vi "RSNRPZ Configure Statistics Scale.vi"(6 "Range (50.0)":dbl=50.0 format="%^.3e", 7 "Points (200)":i32=200, 8 "error in (no error)":errorcluster, 9 "Reference Level (-30.0 dB)":dbl=-30.0 format="%^.3e", 10 "Channel (1)":i32=1, 11 "VISA session":refnum<visa-resource-name> caption="VISA resource name") -> (0 "error out":errorcluster, 3 "dup VISA session":refnum<visa-resource-name> caption="VISA resource name")   [LabVIEW 2010]
doc: "This VI sets the X-Axis of statistical measurement.\n\nRemote-control command(s):\nSENSe:STATistics:SCALE:X:RLEVel\nSENSe:STATistics:SCALE:X:RANGe\nSENSe:STATistics:SCALE:X:POINts"
uses:
  rsnrpz_32.dll
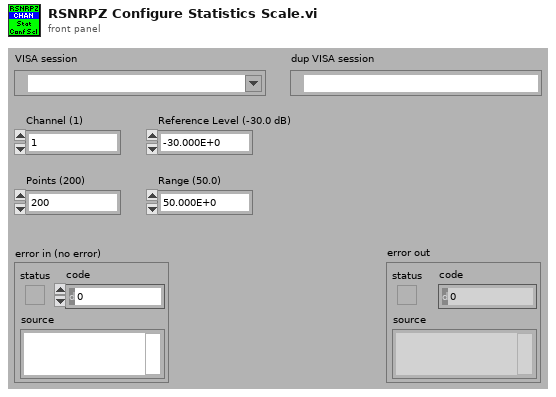
[diagram p1: front panel]
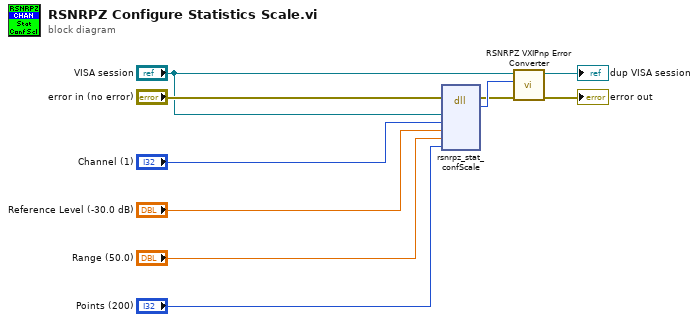
[diagram p0: block diagram]
diagram:
  n1 = dll-call lib="rsnrpz_32.dll" fn="rsnrpz_stat_confScale"(error in="error in (no error)", "Instrument Handle"="VISA session", "Channel"="Channel (1)", "Reference Level"="Reference Level (-30.0 dB)", "Range"="Range (50.0)", "Points"="Points (200)") -> (error out=w5:errorcluster, "Status"=w10:i32)  [unwired: 7 in, 1 out]
  n2 = call <instrlib>:"RSNRPZ VXIPnp Error Converter.vi"("error in"=w5, "VXIPnp error code"=w10, "VISA session"="VISA session") -> ("error out"=→"error out":errorcluster, "dup VISA session"=→"dup VISA session":refnum<visa-resource-name>)  [unwired: 7 in]
